vi "HFRR ADV v03 new software.vi"() -> ()   [LabVIEW 2025] (continued)
                frame 126, Default {
                }
              }
            }
          }
          frame #1 {
            w4146 = TRUE ("Visible")
            n3112 = local read "S 91"() -> (w4163:string)
            n3113 = local read "S 90"() -> (w4162:string)
            n3114 = local read "S 88"() -> (w4161:string)
            n3115 = property on="File Path" class="Path"("Caption.Text"=w4162) -> ()  [unwired: 2 in, 2 out]
            n3116 = property on="SrvM CP" class="Bool (strict)"("Boolean Text.Text"=w4161) -> ()  [unwired: 2 in, 2 out]
            n3117 = local read "S 71"() -> (w4156:string)
            n3118 = local read "S 86"() -> (w4158:string)
            n3119 = local read "S 85"() -> (w4159:string)
            n3120 = local read "S 87"() -> (w4157:string)
            n3121 = local read "S 84"() -> (w4160:string)
            n3122 = local read "S 103"() -> (w4145:string)
            n3123 = local read "S 104"() -> (w4144:string)
            n3124 = property on="ENTER THE NEW PASSWORD" class="Str"("Caption.Text"=w4157) -> ()  [unwired: 2 in, 2 out]
            n3125 = property on="Password" class="Str"("Caption.Text"=w4159) -> ()  [unwired: 2 in, 2 out]
            n3126 = property on="ENTER CURRENT PASSWORD" class="Str"("Caption.Text"=w4158) -> ()  [unwired: 2 in, 2 out]
            n3127 = property on="EDIT" class="Bool (strict)"("Boolean Text.Text"=w4156) -> ()  [unwired: 2 in, 2 out]
            n3128 = property on="SAVE" class="Bool (strict)"("Boolean Text.Text"=w4160) -> ()  [unwired: 2 in, 2 out]
            n3129 = Build Array(w4145, w4144) -> (w4143:string[])
            n3130 = property on="Heater Button" class="Bool (strict)"("Strings [4]"=w4143) -> ()  [unwired: 2 in, 2 out]
            n3131 = property on="CH-HUMIDITY WET" class="DigNum (strict)"("Caption.Size to Text?"=w4146) -> ()  [unwired: 2 in, 2 out]
            n3132 = property on="CH-HUMIDITY DRY" class="DigNum (strict)"("Caption.Size to Text?"=w4146) -> ()  [unwired: 2 in, 2 out]
            n3133 = property on="CH-POWER -" class="DigNum (strict)"("Caption.Size to Text?"=w4146) -> ()  [unwired: 2 in, 2 out]
            n3134 = property on="CH-HEATER" class="DigNum (strict)"("Caption.Size to Text?"=w4146) -> ()  [unwired: 2 in, 2 out]
            n3135 = property on="CH-POWER +" class="DigNum (strict)"("Caption.Size to Text?"=w4146) -> ()  [unwired: 2 in, 2 out]
            n3136 = local read "S 92"() -> (w4155:string)
            n3137 = local read "S 93"() -> (w4154:string)
            n3138 = local read "S 105"() -> (w4141:string)
            n3139 = local read "S 106"() -> (w4140:string)
            n3140 = Build Array(w4155, w4154) -> ()  [unwired: 1 out]
            n3141 = Build Array(w4141, w4140) -> (w4142:string[])
            n3142 = local read "S 95"() -> (w4152:string)
            n3143 = local read "S 94"() -> (w4153:string)
            n3144 = local read "bs"() -> (w4168:string)
            n3145 = local read "as"() -> (w4169:string)
            n3146 = property on="Humidity" class="Bool (strict)"("Strings [4]"=w4142) -> ()  [unwired: 2 in, 2 out]
            n3147 = Concatenate Strings(w4168, "\r", w4169) -> ()  [unwired: 1 out]
            n3148 = property on="STROKE GAIN :" class="DigNum (strict)"("Caption.Text"=w4152) -> ()  [unwired: 2 in, 2 out]
            n3149 = property on="DISPLACEMENT :" class="DigNum (strict)"("Caption.Text"=w4153) -> ()  [unwired: 2 in, 2 out]
            n3150 = property on="Rh After" class="DigNum (strict)"("Caption.Size to Text?"=TRUE ("Caption.Size to Text")) -> ()  [unwired: 2 in, 2 out]
            n3151 = local read "S 48"() -> (w4192:string)
            n3152 = local read "S 50"() -> (w4190:string)
            n3153 = local read "S 51"() -> (w4189:string)
            n3154 = local read "S 49"() -> (w4191:string)
            n3155 = local read "S 52"() -> (w4188:string)
            n3156 = local read "as"() -> (w4173:string)
            n3157 = local read "bs"() -> (w4174:string)
            n3158 = local read "S 56"() -> (w4187:string)
            n3159 = local read "S 57"() -> (w4186:string)
            n3160 = local read "S 58"() -> (w4185:string)
            n3161 = local read "S 59"() -> (w4184:string)
            n3162 = property on="OPEN" class="Bool (strict)"("Boolean Text.Text"=w4188) -> ()  [unwired: 2 in, 2 out]
            n3163 = property on="OPEN 1" class="Bool (strict)"("Boolean Text.Text"=w4192) -> ()  [unwired: 2 in, 2 out]
            n3164 = property on="OPEN 2" class="Bool (strict)"("Boolean Text.Text"=w4191) -> ()  [unwired: 2 in, 2 out]
            n3165 = property on="OPEN 3" class="Bool (strict)"("Boolean Text.Text"=w4190) -> ()  [unwired: 2 in, 2 out]
            n3166 = property on="OPEN 4" class="Bool (strict)"("Boolean Text.Text"=w4189) -> ()  [unwired: 2 in, 2 out]
            n3167 = Concatenate Strings(w4174, "\r", w4173) -> ()  [unwired: 1 out]
            n3168 = local read "S 102"() -> (w4147:string)
            n3169 = property on="КОФ1" class="DigNum (strict)"("Caption.Text"=w4187) -> ()  [unwired: 2 in, 2 out]
            n3170 = local read "S 98"() -> (w4151:string)
            n3171 = local read "S 99"() -> (w4150:string)
            n3172 = local read "S 100"() -> (w4149:string)
            n3173 = local read "S 101"() -> (w4148:string)
            n3174 = property on="КОФ2" class="DigNum (strict)"("Caption.Text"=w4186) -> ()  [unwired: 2 in, 2 out]
            n3175 = property on="КОФ3" class="DigNum (strict)"("Caption.Text"=w4185) -> ()  [unwired: 2 in, 2 out]
            n3176 = property on="КОФ4" class="DigNum (strict)"("Caption.Text"=w4184) -> ()  [unwired: 2 in, 2 out]
            n3177 = local read "bs"() -> (w4172:string)
            n3178 = local read "as"() -> (w4171:string)
            n3179 = property on="CH-POWER +" class="DigNum (strict)"("Caption.Text"=w4151) -> ()  [unwired: 2 in, 2 out]
            n3180 = property on="CH-POWER -" class="DigNum (strict)"("Caption.Text"=w4150) -> ()  [unwired: 2 in, 2 out]
            n3181 = property on="CH-HEATER" class="DigNum (strict)"("Caption.Text"=w4149) -> ()  [unwired: 2 in, 2 out]
            n3182 = property on="CH-HUMIDITY DRY" class="DigNum (strict)"("Caption.Text"=w4148) -> ()  [unwired: 2 in, 2 out]
            n3183 = property on="CH-HUMIDITY WET" class="DigNum (strict)"("Caption.Text"=w4147) -> ()  [unwired: 2 in, 2 out]
            n3184 = local read "S 60"() -> (w4183:string)
            n3185 = local read "S 54"() -> (w4193:string)
            n3186 = Concatenate Strings(w4172, "\r", w4171) -> ()  [unwired: 1 out]
            n3187 = Concatenate Strings(w4193, w4183) -> ()  [unwired: 1 out]
            n3188 = local read "S 77"() -> (→"String 43":string)
            n3189 = local read "S 76"() -> (w4166:string)
            n3190 = local read "S 78"() -> (w4165:string)
            n3191 = local read "S 71"() -> (w4177:string)
            n3192 = local read "S 66"() -> (w4182:string)
            n3193 = local read "S 67"() -> (w4181:string)
            n3194 = local read "S 68"() -> (w4180:string)
            n3195 = local read "S 69"() -> (w4179:string)
            n3196 = local read "S 70"() -> (w4178:string)
            n3197 = property on="AIR TEMP" class="DigNum (strict)"("Caption.Text"=w4165) -> ()  [unwired: 2 in, 2 out]
            n3198 = property on="Set Strk" class="DigNum (strict)"("Caption.Text"=w4166) -> ()  [unwired: 2 in, 2 out]
            n3199 = property on="FRIC. FORCE :" class="DigNum (strict)"("Caption.Text"=w4182) -> ()  [unwired: 2 in, 2 out]
            n3200 = property on="TEMPERATURE :" class="DigNum (strict)"("Caption.Text"=w4181) -> ()  [unwired: 2 in, 2 out]
            n3201 = property on="SPEED OUT:" class="DigNum (strict)"("Caption.Text"=w4180) -> ()  [unwired: 2 in, 2 out]
            n3202 = property on="AIR TEMPERATURE :" class="DigNum (strict)"("Caption.Text"=w4179) -> ()  [unwired: 2 in, 2 out]
            n3203 = property on="HUMIDITY:" class="DigNum (strict)"("Caption.Text"=w4178) -> ()  [unwired: 2 in, 2 out]
            n3204 = property on="EDIT" class="Bool (strict)"("Boolean Text.Text"=w4177) -> ()  [unwired: 2 in, 2 out]
            n3205 = local read "S 79"() -> (w4164:string)
          }
          frame #2 {
          }
        }
        n3206 = local write "Lan flag"(10.0 ("Lan flag")) -> ()
      }
      frame Enabled {
      }
    }
    n3207 = Wait (ms)(milliseconds to wait=u32 2000) -> ()  [unwired: 1 out]
    n3208 = local read "Quit"() -> (w3967:bool)
  }
  n3209 = disable-structure shown="Disabled" {
    frame Disabled {
      n3210 = while {
        tunnel: [w4195] -> _
        i -> [w4195]
        stop <- w4194 continue-if-true
        n3211 = Wait (ms)(milliseconds to wait=u32 50) -> ()  [unwired: 1 out]
        n3212 = stacked-sequence {
          frame #0 {
            # "Controls Text color"
            # "Controls BG color"
            n3213 = property on="FILE" class="Str"("Text.Text Colors:Text Color"="SC  Text") -> ()  [unwired: 2 in, 2 out]
            n3214 = property on="Fuel Discription :" class="Str"("Text.Text Colors:Text Color"="SC  Text") -> ()  [unwired: 2 in, 2 out]
            n3215 = property on="tested by" class="Str"("Text.Text Colors:Text Color"="SC  Text") -> ()  [unwired: 2 in, 2 out]
            n3216 = property on="Remarks :" class="Str"("Text.Text Colors:Text Color"="SC  Text") -> ()  [unwired: 2 in, 2 out]
            n3217 = property class="DigNum (strict)"("Numeric Text.Text Colors:BG Color"="NC BG") -> ()  [unwired: 2 in, 2 out]
            n3218 = property class="DigNum (strict)"("Numeric Text.Text Colors:BG Color"="NC BG") -> ()  [unwired: 2 in, 2 out]
            n3219 = property class="DigNum (strict)"("Numeric Text.Text Colors:BG Color"="NC BG") -> ()  [unwired: 2 in, 2 out]
            n3220 = property class="DigNum (strict)"("Numeric Text.Text Colors:BG Color"="NC BG") -> ()  [unwired: 2 in, 2 out]
            n3221 = property class="DigNum (strict)"("Numeric Text.Text Colors:BG Color"="NC BG") -> ()  [unwired: 2 in, 2 out]
            n3222 = property class="DigNum (strict)"("Numeric Text.Text Colors:BG Color"="NC BG") -> ()  [unwired: 2 in, 2 out]
            n3223 = property class="DigNum (strict)"("Numeric Text.Text Colors:BG Color"="NC BG") -> ()  [unwired: 2 in, 2 out]
            n3224 = property class="DigNum (strict)"("Numeric Text.Text Colors:BG Color"="NC BG") -> ()  [unwired: 2 in, 2 out]
            n3225 = property class="DigNum (strict)"("Numeric Text.Text Colors:BG Color"="NC BG") -> ()  [unwired: 2 in, 2 out]
            n3226 = property class="DigNum (strict)"("Numeric Text.Text Colors:BG Color"="NC BG") -> ()  [unwired: 2 in, 2 out]
            n3227 = property class="DigNum (strict)"("Numeric Text.Text Colors:BG Color"="NC BG") -> ()  [unwired: 2 in, 2 out]
            n3228 = property class="DigNum (strict)"("Numeric Text.Text Colors:BG Color"="NC BG") -> ()  [unwired: 2 in, 2 out]
            n3229 = property on="FILE" class="Str"("Text.Text Colors:BG Color"="SC BG 3") -> ()  [unwired: 2 in, 2 out]
            n3230 = property on="Fuel Discription :" class="Str"("Text.Text Colors:BG Color"="SC BG 3") -> ()  [unwired: 2 in, 2 out]
            n3231 = property on="tested by" class="Str"("Text.Text Colors:BG Color"="SC BG 3") -> ()  [unwired: 2 in, 2 out]
            n3232 = property on="Remarks :" class="Str"("Text.Text Colors:BG Color"="SC BG 3") -> ()  [unwired: 2 in, 2 out]
            n3233 = property class="DigNum (strict)"("Numeric Text.Text Colors:Text Color"="NC Text") -> ()  [unwired: 2 in, 2 out]
            n3234 = property class="DigNum (strict)"("Numeric Text.Text Colors:Text Color"="NC Text") -> ()  [unwired: 2 in, 2 out]
            n3235 = property class="DigNum (strict)"("Numeric Text.Text Colors:Text Color"="NC Text") -> ()  [unwired: 2 in, 2 out]
            n3236 = property class="DigNum (strict)"("Numeric Text.Text Colors:Text Color"="NC Text") -> ()  [unwired: 2 in, 2 out]
            n3237 = property class="DigNum (strict)"("Numeric Text.Text Colors:Text Color"="NC Text") -> ()  [unwired: 2 in, 2 out]
            n3238 = property class="DigNum (strict)"("Numeric Text.Text Colors:Text Color"="NC Text") -> ()  [unwired: 2 in, 2 out]
            n3239 = property class="DigNum (strict)"("Numeric Text.Text Colors:Text Color"="NC Text") -> ()  [unwired: 2 in, 2 out]
            n3240 = property class="DigNum (strict)"("Numeric Text.Text Colors:Text Color"="NC Text") -> ()  [unwired: 2 in, 2 out]
            n3241 = property class="DigNum (strict)"("Numeric Text.Text Colors:Text Color"="NC Text") -> ()  [unwired: 2 in, 2 out]
            n3242 = property class="DigNum (strict)"("Numeric Text.Text Colors:Text Color"="NC Text") -> ()  [unwired: 2 in, 2 out]
            n3243 = property class="DigNum (strict)"("Numeric Text.Text Colors:Text Color"="NC Text") -> ()  [unwired: 2 in, 2 out]
            n3244 = property class="DigNum (strict)"("Numeric Text.Text Colors:Text Color"="NC Text") -> ()  [unwired: 2 in, 2 out]
            n3245 = property class="DigNum (strict)"("Numeric Text.Text Colors:Text Color"="NI Text  2") -> ()  [unwired: 2 in, 2 out]
            n3246 = property class="DigNum (strict)"("Numeric Text.Text Colors:Text Color"="NI Text  2") -> ()  [unwired: 2 in, 2 out]
            n3247 = property class="DigNum (strict)"("Numeric Text.Text Colors:Text Color"="NI Text  2") -> ()  [unwired: 2 in, 2 out]
            n3248 = property class="DigNum (strict)"("Numeric Text.Text Colors:Text Color"="NI Text  2") -> ()  [unwired: 2 in, 2 out]
            n3249 = property class="DigNum (strict)"("Numeric Text.Text Colors:Text Color"="NI Text  2") -> ()  [unwired: 2 in, 2 out]
            n3250 = property class="DigNum (strict)"("Numeric Text.Text Colors:Text Color"="NI Text  2") -> ()  [unwired: 2 in, 2 out]
            n3251 = property class="DigNum (strict)"("Numeric Text.Text Colors:Text Color"="NI Text  2") -> ()  [unwired: 2 in, 2 out]
            n3252 = property class="DigNum (strict)"("Numeric Text.Text Colors:Text Color"="NI Text  2") -> ()  [unwired: 2 in, 2 out]
            n3253 = property class="DigNum (strict)"("Numeric Text.Text Colors:Text Color"="NI Text  2") -> ()  [unwired: 2 in, 2 out]
            n3254 = property class="DigNum (strict)"("Numeric Text.Text Colors:Text Color"="NI Text  2") -> ()  [unwired: 2 in, 2 out]
            n3255 = property class="DigNum (strict)"("Numeric Text.Text Colors:Text Color"="NI Text  2") -> ()  [unwired: 2 in, 2 out]
            n3256 = property class="DigNum (strict)"("Numeric Text.Text Colors:Text Color"="NI Text  2") -> ()  [unwired: 2 in, 2 out]
            n3257 = property class="DigNum (strict)"("Numeric Text.Text Colors:Text Color"="NI Text  2") -> ()  [unwired: 2 in, 2 out]
            n3258 = property class="DigNum (strict)"("Numeric Text.Text Colors:Text Color"="NI Text  2") -> ()  [unwired: 2 in, 2 out]
            n3259 = property class="DigNum (strict)"("Numeric Text.Text Colors:Text Color"="NI Text  2") -> ()  [unwired: 2 in, 2 out]
            n3260 = property on="Coefficient Of Friction" class="XYGraph (strict)"("Plot Area:Colors:FG Color"="GFG  2", "Plot Area:Colors:BG Color"="GBG   2") -> ()  [unwired: 2 in, 2 out]
            n3261 = property on="Humidity ( %RH )" class="XYGraph (strict)"("Plot Area:Colors:FG Color"="GFG  2", "Plot Area:Colors:BG Color"="GBG   2") -> ()  [unwired: 2 in, 2 out]
            n3262 = property on="Air Temperature  ( °C )" class="XYGraph (strict)"("Plot Area:Colors:FG Color"="GFG  2", "Plot Area:Colors:BG Color"="GBG   2") -> ()  [unwired: 2 in, 2 out]
            n3263 = property on="Sample Temperature ( °C )" class="XYGraph (strict)"("Plot Area:Colors:FG Color"="GFG  2", "Plot Area:Colors:BG Color"="GBG   2") -> ()  [unwired: 2 in, 2 out]
            n3264 = property class="DigNum (strict)"("Numeric Text.Text Colors:BG Color"="NI BG 2") -> ()  [unwired: 2 in, 2 out]
            n3265 = property class="DigNum (strict)"("Numeric Text.Text Colors:BG Color"="NI BG 2") -> ()  [unwired: 2 in, 2 out]
            n3266 = property class="DigNum (strict)"("Numeric Text.Text Colors:BG Color"="NI BG 2") -> ()  [unwired: 2 in, 2 out]
            n3267 = property class="DigNum (strict)"("Numeric Text.Text Colors:BG Color"="NI BG 2") -> ()  [unwired: 2 in, 2 out]
            n3268 = property class="DigNum (strict)"("Numeric Text.Text Colors:BG Color"="NI BG 2") -> ()  [unwired: 2 in, 2 out]
            n3269 = property class="DigNum (strict)"("Numeric Text.Text Colors:BG Color"="NI BG 2") -> ()  [unwired: 2 in, 2 out]
            n3270 = property class="DigNum (strict)"("Numeric Text.Text Colors:BG Color"="NI BG 2") -> ()  [unwired: 2 in, 2 out]
            n3271 = property class="DigNum (strict)"("Numeric Text.Text Colors:BG Color"="NI BG 2") -> ()  [unwired: 2 in, 2 out]
            n3272 = property class="DigNum (strict)"("Numeric Text.Text Colors:BG Color"="NI BG 2") -> ()  [unwired: 2 in, 2 out]
            n3273 = property class="DigNum (strict)"("Numeric Text.Text Colors:BG Color"="NI BG 2") -> ()  [unwired: 2 in, 2 out]
            n3274 = property class="DigNum (strict)"("Numeric Text.Text Colors:BG Color"="NI BG 2") -> ()  [unwired: 2 in, 2 out]
            n3275 = property class="DigNum (strict)"("Numeric Text.Text Colors:BG Color"="NI BG 2") -> ()  [unwired: 2 in, 2 out]
            n3276 = property class="DigNum (strict)"("Numeric Text.Text Colors:BG Color"="NI BG 2") -> ()  [unwired: 2 in, 2 out]
            n3277 = property class="DigNum (strict)"("Numeric Text.Text Colors:BG Color"="NI BG 2") -> ()  [unwired: 2 in, 2 out]
            n3278 = property class="DigNum (strict)"("Numeric Text.Text Colors:BG Color"="NI BG 2") -> ()  [unwired: 2 in, 2 out]
            n3279 = property class="Bool"("Colors [4]"="Boolean BC T & BG") -> ()  [unwired: 2 in, 2 out]
            n3280 = property on="Save & Continue" class="Bool (strict)"("Colors [4]"="Boolean BC T & BG") -> ()  [unwired: 2 in, 2 out]
            n3281 = property on="Heater Button" class="Bool (strict)"("Colors [4]"="Boolean BC T & BG") -> ()  [unwired: 2 in, 2 out]
            n3282 = property class="Bool"("Colors [4]"="Boolean BC T & BG") -> ()  [unwired: 2 in, 2 out]
            n3283 = property on="Humidity" class="Bool (strict)"("Colors [4]"="Boolean BC T & BG") -> ()  [unwired: 2 in, 2 out]
            n3284 = property class="Bool (strict)"("Colors [4]"="Boolean BC T & BG") -> ()  [unwired: 2 in, 2 out]
            n3285 = property on="RUN" class="Bool (strict)"("Colors [4]"="Boolean BC T & BG") -> ()  [unwired: 2 in, 2 out]
            n3286 = property on="trip1 8" class="Bool (strict)"("Colors [4]"="Boolean BC T & BG") -> ()  [unwired: 2 in, 2 out]
            n3287 = property class="Bool"("Colors [4]"="Boolean BC T & BG") -> ()  [unwired: 2 in, 2 out]
            n3288 = property class="Bool (strict)"("Colors [4]"="Boolean BC T & BG") -> ()  [unwired: 2 in, 2 out]
            n3289 = property on="OPEN 1" class="Bool (strict)"("Colors [4]"="Boolean BC T & BG 2") -> ()  [unwired: 2 in, 2 out]
            n3290 = property on="OPEN 2" class="Bool (strict)"("Colors [4]"="Boolean BC T & BG 2") -> ()  [unwired: 2 in, 2 out]
            n3291 = property on="OPEN 3" class="Bool (strict)"("Colors [4]"="Boolean BC T & BG 2") -> ()  [unwired: 2 in, 2 out]
            n3292 = property on="OPEN 4" class="Bool (strict)"("Colors [4]"="Boolean BC T & BG 2") -> ()  [unwired: 2 in, 2 out]
            n3293 = property on="OPEN" class="Bool (strict)"("Colors [4]"="Boolean BC T & BG 2") -> ()  [unwired: 2 in, 2 out]
            n3294 = property on="rstv2" class="Bool"("Colors [4]"="Boolean BC T & BG 2") -> ()  [unwired: 2 in, 2 out]
            n3295 = property on="RST CP" class="Bool"("Colors [4]"="Boolean BC T & BG 2") -> ()  [unwired: 2 in, 2 out]
            n3296 = property on="RSTV1 3" class="Bool"("Colors [4]"="Boolean BC T & BG 2") -> ()  [unwired: 2 in, 2 out]
            n3297 = property on="RSTV1 2" class="Bool"("Colors [4]"="Boolean BC T & BG 2") -> ()  [unwired: 2 in, 2 out]
          }
          frame #1 {
          }
        }
        n3298 = local read "Quit"() -> (w4194:bool)
      }
    }
    frame Enabled {
    }
  }
  n3299 = while {
    shift-right: [w4212] -> _
    shift-left: _ -> [w4213]
    shift-right: [w4210] -> _
    shift-left: T14 {"Read Heave and Surge"="", "Bytes at Heave Port"=0.0, "Heave and Surge COM Port:"="COM9", "Com Port 2"="COM7", "Residual Due"="", "Heave COM Status 2"=TRUE, "Heave COM Status"=TRUE, "Port 2"=TRUE, "Sway PPR"=6400.0, "Surge PPR"=6400.0, "Heave PPR"=6400.0, "Sway Pitch"=2.0, "Surge Pitch"=3.0, "Heave Pitch"=4.0, "Sway Pulses/mm"=320.0, "Surge Pulses/mm"=1600.0, "Heave Pulses/mm"=1600.0, "inner loop"=0.0, "Read Heave and Surge 2"="", "String 36"="", "Write S"=FALSE, "WriteCC1"=[""], "Heave COM Loop"=0, "LastCom"="", "EXIT"=FALSE, "Error Heave"={"status"=TRUE, "code"=-1073807343, "source"=""}} -> [w4209]
    shift-right: [w4207] -> _
    shift-left: enum16{"init", "MAIN", "Panel Close"}."init" -> [w4208]
    stop <- w4211 stop-if-true
    n3300 = case shown="\"init\"" w4208 {
      tunnel: w4213 -> [w4227 w4242 w4312 w4314]
      tunnel: [w4221 w4260 w4312 w4314] -> w4212
      tunnel: [_ _ TRUE _] -> w4211
      tunnel: [w4217 w4257 w4310 w4313] -> w4210
      tunnel: w4209 -> [w4224 w4241 w4310 w4313]
      tunnel: [enum16{"init", "MAIN", "Panel Close"}."MAIN" w4235 _ _] -> w4207
      frame "init" {
        n3301 = Bundle By Name(cluster=w4224, "Heave and Surge COM Port:"="C3 :") -> (w4223:T14)
        n3302 = call "Instrument fgv.vi"("Enum"=T24."INIT", "error in (no error) 2"=w4227, "INPUT"=w4223) -> ("error"=w4225:errorcluster, "output"=w4220:T14)  [unwired: 6 in, 1 out]
        n3303 = case shown="No Error" w4225 {
          selector: w4225 -> [w4229 _]
          tunnel: [w4229 w4233] -> w4221
          tunnel: w4220 -> [w4228 w4231]
          tunnel: [w4228 w4230] -> w4218
          frame No Error {
          }
          frame Error {
            n3304 = call "Instrument fgv.vi"("Enum"=T24."ERROR INIT", "INPUT"=w4231) -> ("error"=w4234:errorcluster, "output"=w4230:T14)  [unwired: 7 in, 1 out]
            n3305 = call <vilib>:"Clear Errors.vi"("error in (no error)"=w4234) -> ("error out"=w4233:errorcluster)  [unwired: 5 in, 1 out]
          }
        }
        n3306 = local read "LastCom"() -> (w4216:string)
        n3307 = Unbundle By Name(w4218) -> ("Heave COM Status 2"=→"COM Status" →"Instrument Status":bool, "Error Heave"=→"Error":errorcluster)  [unwired: 1 out]
        n3308 = Bundle By Name(cluster=w4218, "LastCom"=w4216) -> (w4217:T14)
      }
      frame "MAIN" {
        n3309 = Unbundle By Name(w4241) -> ("Com Port 2"=w4262:refnum<visa-resource-name>)
        n3310 = local write "Com Port 4"(w4262) -> ()
        n3311 = local read "C3 :"() -> (w4239:refnum<visa-resource-name>)
        n3312 = Divide(x="Heave PPR", y="Heave Pitch") -> (x/y=→"Heave Pulses/mm":dbl)
        n3313 = Bundle By Name(cluster=w4241, "Heave and Surge COM Port:"=w4239) -> (w4240:T14)
        n3314 = Equal?(x=w4262, y=w4239) -> (x = y?=w4261:bool)
        n3315 = Divide(x="Sway PPR", y="Sway Pitch") -> (x/y=→"Sway Pulses/mm":dbl)
        n3316 = case shown="False" w4261 {
          tunnel: [w4266 w4283] -> w4260
          tunnel: w4242 -> [w4267 w4289]
          tunnel: w4240 -> [w4265 w4287]
          tunnel: [w4264 w4282] -> w4257
          frame False {
            n3317 = call <vilib>:"Clear Errors.vi"("error in (no error)"=w4267) -> ("error out"=w4263:errorcluster)  [unwired: 5 in, 1 out]
            n3318 = call "Instrument fgv.vi"("Enum"=T24."ERROR INIT", "error in (no error) 2"=w4263, "INPUT"=w4265) -> ("error"=w4269:errorcluster, "output"=w4264:T14)  [unwired: 6 in, 1 out]
            n3319 = call <vilib>:"Clear Errors.vi"("error in (no error)"=w4269) -> ("error out"=w4266:errorcluster)  [unwired: 5 in, 1 out]
          }
          frame True {
            n3320 = call "Instrument fgv.vi"("Enum"=T24."READ", "error in (no error) 2"=w4289, "INPUT"=w4287) -> ("error"=w4288:errorcluster, "output"=w4279:T14)  [unwired: 6 in, 1 out]
            n3321 = Bundle By Name(cluster=w4279, "String 36"="String 11") -> (w4278:T14)
            n3322 = case shown="True" "Write S" {
              selector: "Write S" -> [_ w4309]
              tunnel: w4288 -> [w4302 w4308]
              tunnel: [w4302 w4307] -> w4275
              tunnel: w4278 -> [w4301 w4304]
              tunnel: [w4301 w4303] -> w4274
              frame False {
              }
              frame True {
                n3323 = Not(x=w4309) -> (.not. x?=w4305:bool)
                n3324 = local write "Write S"(w4305) -> ()
                n3325 = call "Instrument fgv.vi"("Enum"=T24."MANUAL WRITE", "error in (no error) 2"=w4308, "INPUT"=w4304) -> ("error"=w4307:errorcluster, "output"=w4303:T14)  [unwired: 6 in, 1 out]
              }
            }
            n3326 = Array Size(array="WriteHumidity") -> (size(s)=w4272:i32)
            n3327 = Greater Than 0?(x=w4272) -> (x > 0?=w4270:bool)
            n3328 = call "Instrument fgv.vi"("Enum"=T24."WRITE", "error in (no error) 2"=w4275, "WriteCC1"="WriteHumidity", "INPUT"=w4274) -> ("error"=w4285:errorcluster, "WriteCC1 2"=w4273:string[], "output"=w4284:T14)  [unwired: 5 in]
            n3329 = case shown="True" w4270 {
              tunnel: w4273 -> [_ w4291]
              frame False {
              }
              frame True {
                n3330 = local write "WriteHumidity"(w4291) -> ()
              }
            }
            n3331 = case shown="Error" w4285 {
              selector: w4285 -> [w4292 w4295]
              tunnel: w4284 -> [w4293 w4300]
              tunnel: [w4293 w4299] -> w4282
              tunnel: [w4292 w4297] -> w4283
              frame No Error {
              }
              frame Error {
                n3332 = call <vilib>:"Clear Errors.vi"("error in (no error)"=w4295) -> ("error out"=w4294:errorcluster)  [unwired: 5 in, 1 out]
                n3333 = call "Instrument fgv.vi"("Enum"=T24."ERROR INIT", "error in (no error) 2"=w4294, "INPUT"=w4300) -> ("error"=w4298:errorcluster, "output"=w4299:T14)  [unwired: 6 in, 1 out]
                n3334 = call <vilib>:"Clear Errors.vi"("error in (no error)"=w4298) -> ("error out"=w4297:errorcluster)  [unwired: 5 in, 1 out]
              }
            }
            n3335 = Unbundle By Name(w4282) -> ("LastCom"=→"LastCom":string, "Read Heave and Surge"=→"Read Humidity":string)
          }
        }
        n3336 = Divide(x="Surge PPR", y="Surge Pitch") -> (x/y=→"Surge Pulses/mm":dbl)
        n3337 = Unbundle By Name(w4257) -> ("Heave COM Status 2"=w4259:bool, "Heave COM Status"=w4258:bool, "Error Heave"=w4255:errorcluster, "Bytes at Heave Port"=→"Bytes at Humidity Port":dbl)
        n3338 = Unbundle By Name(w4255) -> ("status"=→"Humidity Port":bool)
        n3339 = Not(x=w4258) -> (.not. x?=w4243:bool)
        n3340 = local write "Error"(w4255) -> ()
        n3341 = Not(x=w4259) -> (.not. x?=w4244:bool)
        n3342 = local write "Instrument Status"(w4243) -> ()
        n3343 = local write "COM Status"(w4244) -> ()
        n3344 = local read "Quit"() -> (w4236:bool)
        n3345 = Select(t=enum16{"init", "MAIN", "Panel Close"}."Panel Close", s=w4236, f=enum16{"init", "MAIN", "Panel Close"}."MAIN") -> (s? t:f=w4235:enum16{"init", "MAIN", "Panel Close"})
      }
      frame "Panel Close" {
      }
      frame Default {
      }
    }
  }
  n3346 = while {
    stop <- w4340 stop-if-true
    n3347 = local read "Read Humidity"() -> (w4321:string)
    n3348 = call <vilib>:"High Resolution Polling Wait.vi"("seconds to wait"=0.1) -> ()  [unwired: 10 in, 1 out]
    n3349 = Spreadsheet String To Array(delimiter (Tab)=",", format string="", spreadsheet string=w4321, array type (2D Dbl)=string[] []) -> (array=w4335:string[])
    n3350 = for {
      tunnel: w4335 -> [w4345] mode=indexing
      tunnel: string[] ["STATE;", "SET;", "RH;", "T;", "AMB_RH;", "AMB_T;", "PUMP;", "FAN_IN;", "FAN_OUT;", "DEHUM;", "CURRENT;", "STALL;"] -> [w4344] mode=indexing
      tunnel: [w4343] -> w4334 mode=indexing
      n3351 = Match Pattern(string=w4345, regular expression=w4344) -> (after substring=w4343:string)  [unwired: 1 in, 3 out]
    }
    n3352 = Index Array(array=w4334) -> (element #1=→"STATE :":string, element #2=→"SET :":string, element #3=w4323:string, element #4=→"T :":string, element #5=w4320:string, element #6=→"AMB_T :":string, element #7=→"PUMP :":string, element #8=→"FAN_IN :":string, element #9=→"FAN_OUT :":string, element #10=→"DEHUM :":string, element #11=→"CURRENT :":string, element #12=→"STALL :":string)  [unwired: 12 in]
    "RH :" <- w4323
    "AMB_RH :" <- w4320
    n3353 = Fract/Exp String To Number(string=w4323) -> (number=w4315:dbl)  [unwired: 3 in, 1 out]
    n3354 = Fract/Exp String To Number(string=w4320) -> (number=w4319:dbl)  [unwired: 3 in, 1 out]
    n3355 = local write "Ambient Humidity :"(w4319) -> ()
    n3356 = Equal?(x=w4315, y=0.0) -> (x = y?=w4317:bool)
    n3357 = case shown="True" w4317 {
      tunnel: [w4341 w4342] -> w4316
      tunnel: w4315 -> [w4341 _]
      frame False {
        (unwired) 0.0
        "Humidity temp" <- w4341
      }
      frame True {
        n3358 = local read "Humidity temp"() -> (w4342:dbl)
      }
    }
    "RH Numeric:" <- w4316
    n3359 = local read "Quit"() -> (w4340:bool)
  }
  n3360 = disable-structure shown="Disabled" {
    frame Disabled {
      n3361 = while {
        tunnel: [w4579] -> _
        i -> [w4579]
        stop <- w4576 stop-if-true
        n3362 = local read "powstat"() -> (w4577:bool)
        n3363 = case shown="True" w4577 {
          frame False {
          }
          frame True {
            n3364 = local read "RUN"() -> (w4580:bool)
            n3365 = case shown="True" w4580 {
              frame False {
                w4610 = 65.0 ("y")
                n3366 = local read "Set Hz"() -> (w4638:dbl)
                n3367 = local read "NORMAL LOAD"() -> (w4639:dbl)
                n3368 = Multiply(x=w4638, y=60.0) -> (x*y=w4645:dbl)
                n3369 = Multiply(x=1.2 ("y"), y=0.949) -> (x*y=w4614:dbl)
                n3370 = Multiply(x=1.2 ("y"), y=0.8166) -> (x*y=w4618:dbl)
                n3371 = Multiply(x=1.2 ("y"), y=0.851) -> (x*y=w4613:dbl)
                n3372 = local read "FF 2"() -> (w4637:dbl)
                n3373 = Absolute Value(x=w4645) -> (abs(x)=w4643:dbl)
                n3374 = case shown="13.." w4637 {
                  tunnel: [1 2 3] -> w4635
                  frame 0..10, Default {
                    # "Normal"
                  }
                  frame 11, 12 {
                  }
                  frame 13.. {
                  }
                }
                "FF STATE" <- w4635
                n3375 = local read "TEMP"() -> (w4598:dbl)
                n3376 = local read item#-1() -> (w4612)
                n3377 = Less?(x=w4612, y=w4618) -> (x < y?=w4615:bool)
                n3378 = In Range and Coerce(upper limit=w4614, x=w4612, lower limit=w4613) -> (In Range?=w4616:bool)  [unwired: 1 out]
                n3379 = case shown="3601.." w4643 {
                  tunnel: [1 2 3] -> w4641
                  frame 0..3000, Default {
                    # "Normal"
                  }
                  frame 3001..3600 {
                  }
                  frame 3601.. {
                  }
                }
                n3380 = case shown="11.." w4639 {
                  tunnel: [1 3] -> w4640
                  frame 1..10, Default {
                  }
                  frame 11.. {
                  }
                }
                "NL STATE" <- w4640
                n3381 = Multiply(x=1.2 ("y"), y=0.95) -> (x*y=w4628:dbl)
                n3382 = Multiply(x=w4610, y=0.954) -> (x*y=w4602:dbl)
                n3383 = Or(x=w4615, y=w4616) -> (x .or. y?=w4617:bool)
                n3384 = Greater Or Equal?(x=w4612, y=w4628) -> (x >= y?=w4625:bool)
                n3385 = Multiply(x=w4610, y=0.99) -> (x*y=w4599:dbl)
                n3386 = Greater Or Equal?(x=w4598, y=w4599) -> (x >= y?=w4604:bool)
                n3387 = Greater Or Equal?(x=w4598, y=w4602) -> (x >= y?=w4601:bool)
                n3388 = case shown="0, 1, Default" w4612 {
                  tunnel: [1 3] -> w4629
                  frame 0, 1, Default {
                  }
                  frame 2.. {
                  }
                }
                n3389 = case shown="True" w4625 {
                  tunnel: [1 3] -> w4630
                  frame False {
                  }
                  frame True {
                  }
                }
                n3390 = case shown="True" w4617 {
                  tunnel: [1 2] -> w4631
                  frame False {
                  }
                  frame True {
                  }
                }
                n3391 = case shown="..0" w4598 {
                  tunnel: [2 3 3 1] -> w4605
                  frame 61, 62 {
                  }
                  frame 63.. {
                  }
                  frame ..0 {
                  }
                  frame 10..60, Default {
                  }
                }
                n3392 = case shown="True" w4604 {
                  tunnel: [1 3] -> w4606
                  frame False {
                  }
                  frame True {
                  }
                }
                n3393 = Number To Decimal String(number=w4641) -> (decimal integer string=w4642:string)  [unwired: 1 in]
                n3394 = case shown="True" w4601 {
                  tunnel: [1 2] -> w4607
                  frame False {
                  }
                  frame True {
                  }
                }
                n3395 = Number To Decimal String(number=1) -> (decimal integer string=→"Air temp":string)  [unwired: 1 in]
                n3396 = Number To Decimal String(number=w4635) -> (decimal integer string=→"ff_st":string)  [unwired: 1 in]
                n3397 = local write "sp_st"(w4642) -> ()
                n3398 = Number To Decimal String(number=w4640) -> (decimal integer string=→"nl_st":string)  [unwired: 1 in]
                n3399 = Build Array(w4605, w4606, w4607) -> (w4608:i32[])
                n3400 = Build Array(w4629, w4630, w4631) -> (w4632:i32[])
                n3401 = Array Max & Min(array=w4608) -> (max value=w4609:i32)  [unwired: 3 out]
                n3402 = Array Max & Min(array=w4632) -> (max value=w4633:i32)  [unwired: 3 out]
                n3403 = Number To Decimal String(number=w4609) -> (decimal integer string=w4597:string)  [unwired: 1 in]
                n3404 = Number To Decimal String(number=w4633) -> (decimal integer string=→"Stroke Ln 2":string)  [unwired: 1 in]
                n3405 = local write "temp_st"(w4597) -> ()
              }
              frame True {
                w4695 = 65.0 ("y")
                # "Healthy -1\nWarning -2\nError -3"
                n3406 = local read "TEMP"() -> (w4706:dbl)
                n3407 = local read "NORMAL LOAD"() -> (w4710:dbl)
                n3408 = local read "Set Hz"() -> (w4708:dbl)
                n3409 = Multiply(x=1.2 ("y"), y=0.949) -> (x*y=w4690:dbl)
                n3410 = Multiply(x=1.2 ("y"), y=0.8166) -> (x*y=w4686:dbl)
                n3411 = Multiply(x=1.2 ("y"), y=0.851) -> (x*y=w4691:dbl)
                n3412 = Multiply(x=w4695, y=0.954) -> (x*y=w4702:dbl)
                n3413 = Multiply(x=w4695, y=0.99) -> (x*y=w4705:dbl)
                n3414 = Greater Or Equal?(x=w4706, y=w4705) -> (x >= y?=w4700:bool)
                n3415 = Multiply(x=w4708, y=60.0) -> (x*y=w4714:dbl)
                n3416 = Greater Or Equal?(x=w4706, y=w4702) -> (x >= y?=w4703:bool)
                n3417 = local read "FF 2"() -> (w4709:dbl)
                n3418 = local read item#-1() -> (w4692)
                n3419 = Less?(x=w4692, y=w4686) -> (x < y?=w4689:bool)
                n3420 = In Range and Coerce(upper limit=w4690, x=w4692, lower limit=w4691) -> (In Range?=w4688:bool)  [unwired: 1 out]
                n3421 = Absolute Value(x=w4714) -> (abs(x)=w4712:dbl)
                n3422 = case shown="63.." w4706 {
                  tunnel: [2 3 3 1] -> w4699
                  frame 61, 62 {
                  }
                  frame 63.. {
                  }
                  frame ..0 {
                  }
                  frame 10..60, Default {
                  }
                }
                n3423 = case shown="True" w4700 {
                  tunnel: [1 3] -> w4698
                  frame False {
                  }
                  frame True {
                  }
                }
                n3424 = case shown="True" w4703 {
                  tunnel: [1 2] -> w4697
                  frame False {
                  }
                  frame True {
                  }
                }
                n3425 = Multiply(x=1.2 ("y"), y=0.95) -> (x*y=w4676:dbl)
                n3426 = case shown="1..10, Default" w4710 {
                  tunnel: [1 3] -> w4717
                  frame 1..10, Default {
                  }
                  frame 11.. {
                  }
                }
                n3427 = case shown="0..10, Default" w4709 {
                  tunnel: [1 2 3] -> w4716
                  frame 0..10, Default {
                  }
                  frame 11, 12 {
                  }
                  frame 13.. {
                  }
                }
                n3428 = case shown="3601.." w4712 {
                  tunnel: [1 2 3] -> w4711
                  frame 0..3000, Default {
                    # "Normal"
                  }
                  frame 3001..3600 {
                  }
                  frame 3601.. {
                  }
                }
                n3429 = Or(x=w4689, y=w4688) -> (x .or. y?=w4687:bool)
                n3430 = Greater Or Equal?(x=w4692, y=w4676) -> (x >= y?=w4679:bool)
                n3431 = case shown="0, 1, Default" w4692 {
                  tunnel: [1 3] -> w4675
                  frame 0, 1, Default {
                  }
                  frame 2.. {
                  }
                }
                n3432 = case shown="True" w4679 {
                  tunnel: [1 3] -> w4674
                  frame False {
                  }
                  frame True {
                  }
                }
                n3433 = case shown="True" w4687 {
                  tunnel: [1 2] -> w4673
                  frame False {
                  }
                  frame True {
                  }
                }
                n3434 = Build Array(w4699, w4698, w4697) -> (w4696:i32[])
                n3435 = Number To Decimal String(number=w4711) -> (decimal integer string=→"sp_st":string)  [unwired: 1 in]
                n3436 = Array Max & Min(array=w4696) -> (max value=w4693:i32)  [unwired: 3 out]
                "TEMP STATE" <- w4693
                n3437 = Number To Decimal String(number=w4717) -> (decimal integer string=w4720:string)  [unwired: 1 in]
                n3438 = Number To Decimal String(number=w4716) -> (decimal integer string=w4718:string)  [unwired: 1 in]
                n3439 = Number To Decimal String(number=w4693) -> (decimal integer string=→"temp_st":string)  [unwired: 1 in]
                n3440 = Build Array(w4675, w4674, w4673) -> (w4672:i32[])
                n3441 = local write "nl_st"(w4720) -> ()
                n3442 = local write "ff_st"(w4718) -> ()
                n3443 = Number To Decimal String(number=1) -> (decimal integer string=w4715:string)  [unwired: 1 in]
                n3444 = Array Max & Min(array=w4672) -> (max value=w4671:i32)  [unwired: 3 out]
                n3445 = local write "Air temp"(w4715) -> ()
                n3446 = Number To Decimal String(number=w4671) -> (decimal integer string=w4670:string)  [unwired: 1 in]
                n3447 = local write "Stroke Ln 2"(w4670) -> ()
              }
            }
            n3448 = local read "Stroke Ln 2"() -> (w4582:string)
            n3449 = local read "nl_st"() -> (w4588:string)
            n3450 = local read "ff_st"() -> (w4585:string)
            n3451 = local read "sp_st"() -> (w4586:string)
            n3452 = local read "temp_st"() -> (w4587:string)
            n3453 = local read "Air temp"() -> (w4581:string)
            n3454 = Replace Array Subset(array="in", new element #1=w4588, index #1=1 ("index"), new element #2=w4585, index #2=2 ("index"), new element #3=w4587, index #3=3 ("index"), new element #4=w4586, index #4=4 ("index"), new element #5=w4582, index #5=5 ("index"), new element #6=w4581, index #6=6 ("index"), new element #7="Sensor State" ("new element/subarray"), index #7=0 ("index")) -> (→"out":string[])
          }
        }
        n3455 = Wait (ms)(milliseconds to wait=u32 10) -> ()  [unwired: 1 out]
        n3456 = local read "Quit"() -> (w4576:bool)
      }
      n3457 = while {
        stop <- w4551 stop-if-true
        n3458 = local read "run replace"() -> (w4553:bool)
        n3459 = Wait (ms)(milliseconds to wait=u32 100) -> ()  [unwired: 1 out]
        n3460 = Equal?(x="FLAG 2", y=0.0) -> (x = y?=w4554:bool)
        n3461 = case shown="True" w4554 {
          frame False {
          }
          frame True {
            n3462 = local write "FLAG 2"(100.0 ("FLAG 2")) -> ()
            n3463 = call <vilib>:"Read Characters From File.vi"("file path (dialog if empty)"=path "C:/LAB-IQ-NXT/WO 2449 TT.sig", "convert eol? (no:F)"=FALSE ("append to file? (new file:F)")) -> ("character string"=w4557:string)  [unwired: 4 in, 3 out]
            n3464 = call <vilib>:"Read Characters From File.vi"("file path (dialog if empty)"=path "C:/LAB-IQ-NXT/WO 2449 TRH.sig", "convert eol? (no:F)"=FALSE ("append to file? (new file:F)")) -> ("character string"=w4558:string)  [unwired: 4 in, 3 out]
            n3465 = Decimal String To Number(string=w4557) -> (number=w4559:i32)  [unwired: 2 in, 1 out]
            n3466 = local write "Total No. of Tests"(w4559) -> ()
            n3467 = Decimal String To Number(string=w4558) -> (number=w4562:i32)  [unwired: 2 in, 1 out]
            n3468 = local write "SEN.RUN HRS"(w4562) -> ()
          }
        }
        n3469 = case shown="True" w4553 {
          frame False {
          }
          frame True {
            n3470 = Equal?(x="FLAG 4", y=0.0) -> (x = y?=w4566:bool)
            n3471 = case shown="False" w4566 {
              frame False {
                n3472 = Get Date/Time In Seconds() -> (seconds since 1Jan1904=w4572:timestamp)
                n3473 = local read "START 3"() -> (w4570:dbl)
                n3474 = To Double Precision Float(number=w4572) -> (double precision float=w4571:dbl)
                n3475 = Subtract(x=w4571, y=w4570) -> (x-y=→"SENSOR TIME":dbl)
              }
              frame True {
                n3476 = Get Date/Time In Seconds() -> (seconds since 1Jan1904=w4574:timestamp)
                n3477 = local write "FLAG 4"(100.0 ("FLAG")) -> ()
                n3478 = To Double Precision Float(number=w4574) -> (double precision float=→"START 3":dbl)
              }
            }
          }
        }
        n3479 = local read "Quit"() -> (w4551:bool)
      }
      n3480 = while {
        shift-right: [w4351] -> _
        shift-left: _ -> [w4352]
        tunnel: [w4347] -> _
        i -> [w4347]
        stop <- w4346 stop-if-true
        n3481 = Wait (ms)(milliseconds to wait=u32 50 ("Refresh Rate (ms)")) -> ()  [unwired: 1 out]
        n3482 = local read "Json End Flg"() -> (w4348:bool)
        n3483 = Not(x="Upld AR 2") -> ()  [unwired: 1 out]
        n3484 = local read "Upld AR 2"() -> (w4349:bool)
        n3485 = call "Elapsed Time9"("Time Target (s)"="Sen.Upload Rate (s)", "Reset"=FALSE, "Auto Reset"=TRUE) -> ("Time has Elapsed"=w4358:bool)  [unwired: 9 in, 7 out]
        n3486 = Or(x=w4358, y=w4348) -> (x .or. y?=w4354:bool)
        n3487 = case shown="True" w4354 {
          frame False {
          }
          frame True {
            w4450 = "\"SensorName\":\"" ("string")
            w4420 = " \"},{"
            w4445 = "\",\"SensorState\":\""
            w4447 = "\",\"SensorModelNumber\":\"" ("string")
            w4446 = "\",\"SensorRuntimeHours\":\"" ("string")
            n3488 = local read "model num"() -> (w4444:string[])
            n3489 = local read "Sensor name"() -> (w4463:string[])
            n3490 = local read "run"() -> (w4434:string[])
            n3491 = local read "SENSOR TIME"() -> (w4390:dbl)
            n3492 = local read "out"() -> (w4383:string[])
            n3493 = local read "Total No. of Tests"() -> (w4388:dbl)
            n3494 = Select(t=60.0, s="Run test 3", f=3600.0) -> (s? t:f=w4398:dbl)
            n3495 = Index Array(array=w4444, index #1=1 ("index")) -> (element #1=w4443:string, element #2=w4442:string, element #3=w4441:string, element #4=w4440:string, element #5=w4439:string, element #6=w4438:string)  [unwired: 5 in]
            n3496 = Index Array(array=w4434, index #1=1 ("index")) -> (element #1=w4433:string, element #2=w4432:string, element #3=w4431:string, element #4=w4430:string, element #5=w4429:string, element #6=w4428:string)  [unwired: 5 in]
            n3497 = Index Array(array=w4463, index #1=1 ("index")) -> (element #1=w4462:string, element #2=w4461:string, element #3=w4460:string, element #4=w4459:string, element #5=w4449:string, element #6=w4448:string)  [unwired: 5 in]
            n3498 = Index Array(array=w4383, index #1=1 ("index")) -> (element #1=w4415:string, element #2=w4414:string, element #3=w4413:string, element #4=w4412:string, element #5=w4411:string, element #6=w4410:string)  [unwired: 5 in]
            n3499 = local read "SEN.RUN HRS"() -> (w4386:dbl)
            n3500 = Divide(x=w4390, y=w4398) -> (x/y=w4397:dbl)
            n3501 = Increment(x=w4397) -> (x+1=w4393:dbl)
            n3502 = Number To Decimal String(number=w4393) -> (decimal integer string=→"run hrs":string)  [unwired: 1 in]
            n3503 = Divide(x=w4386, y=3600.0 ("f")) -> (x/y=w4381:dbl)
            n3504 = Round To Nearest(number=w4381) -> (nearest integer value=w4379:dbl)
            n3505 = Number To Decimal String(number=w4379) -> (decimal integer string=w4380:string)  [unwired: 1 in]
            n3506 = Number To Decimal String(number=w4388) -> (decimal integer string=w4389:string)  [unwired: 1 in]
            n3507 = local read "Model No"() -> (w4394:string)
            n3508 = local read "UUID"() -> (w4489:string)
            n3509 = local read "Serial No"() -> (w4493:string)
            n3510 = local read "Secret Key"() -> (w4494:string)
            n3511 = Concatenate Strings("\",\"MachineSerialNumber\":\"" ("string"), w4493) -> (w4497:string)
            n3512 = Concatenate Strings("\",\"ModelNumber\":\"" ("string"), w4394) -> (w4395:string)
            n3513 = Concatenate Strings("\",\"MachineRuntimeHours\":\"" ("string"), w4380) -> (w4498:string)
            n3514 = Concatenate Strings("\",\"MachineRuntimeCycles\":\"", w4389) -> (w4491:string)
            n3515 = Concatenate Strings(w4447, w4443) -> (w4477:string)
            n3516 = Concatenate Strings(w4446, w4433) -> (w4478:string)
            n3517 = Concatenate Strings(w4445, w4415) -> (w4476:string)
            n3518 = Concatenate Strings(w4497, w4395, w4498, w4491) -> (w4500:string)
            n3519 = Concatenate Strings(w4447, w4442) -> (w4474:string)
            n3520 = Concatenate Strings(w4446, w4432) -> (w4473:string)
            n3521 = Concatenate Strings(w4445, w4414) -> (w4475:string)
            n3522 = Concatenate Strings(w4447, w4441) -> (w4469:string)
            n3523 = Concatenate Strings(w4446, w4431) -> (w4470:string)
            n3524 = Concatenate Strings(w4445, w4413) -> (w4468:string)
            n3525 = Concatenate Strings(w4447, w4440) -> (w4466:string)
            n3526 = Concatenate Strings(w4446, w4430) -> (w4465:string)
            n3527 = Concatenate Strings(w4445, w4412) -> (w4467:string)
            n3528 = Concatenate Strings(w4477, w4478, w4476) -> (w4479:string)
            n3529 = Concatenate Strings(w4447, w4439) -> (w4456:string)
            n3530 = Concatenate Strings(w4446, w4429) -> (w4457:string)
            n3531 = Concatenate Strings(w4447, w4438) -> (w4453:string)
            n3532 = Concatenate Strings(w4446, w4428) -> (w4452:string)
            n3533 = Concatenate Strings(w4445, w4411) -> (w4455:string)
            n3534 = Concatenate Strings(w4445, w4410) -> (w4454:string)
            n3535 = Concatenate Strings("{\"SecretKey\":\"", w4494, w4500, "\",\"UUID\" : \"", w4489, "\",\"SensorInformation\":", "[{" ("string")) -> (w4427:string)
            n3536 = Concatenate Strings(w4474, w4473, w4475) -> (w4472:string)
            n3537 = Concatenate Strings(w4469, w4470, w4468) -> (w4471:string)
            n3538 = Concatenate Strings(w4466, w4465, w4467) -> (w4464:string)
            n3539 = Concatenate Strings(w4456, w4457, w4455) -> (w4458:string)
            n3540 = Concatenate Strings(w4453, w4452, w4454) -> (w4451:string)
            n3541 = Concatenate Strings(w4450, w4462, w4479, w4420) -> (w4426:string)
            n3542 = Concatenate Strings(w4450, w4461, w4472, w4420) -> (w4425:string)
            n3543 = Concatenate Strings(w4450, w4460, w4471, w4420) -> (w4424:string)
            n3544 = Concatenate Strings(w4450, w4459, w4464, w4420) -> (w4423:string)
            n3545 = Concatenate Strings(w4450, w4449, w4458, w4420) -> (w4422:string)
            n3546 = Concatenate Strings(w4450, w4448, w4451, "\"}" ("string")) -> (w4421:string)
            n3547 = Concatenate Strings(w4427, w4426, w4425, w4424, w4423, w4422, w4421, "]}" ("string")) -> (w4418:string)
            n3548 = local read "SEN.RUN HRS"() -> (w4385:dbl)
            n3549 = disable-structure shown="Disabled" {
              frame Disabled {
                n3550 = local read "state"() -> (w4504:string[])
                n3551 = Delete From Array(array=w4504, index=0) -> (array with subset deleted=w4502:string[])  [unwired: 1 in, 1 out]
                n3552 = for {
                  N: 6 -> [_]
                  tunnel: w4502 -> [w4515] mode=indexing
                  tunnel: [w4514] -> w4501 mode=indexing
                  n3553 = Equal?(x=w4515, y="Warning") -> (x = y?=w4511:bool)
                  n3554 = Equal?(x=w4515, y="Healthy") -> (x = y?=w4508:bool)
                  n3555 = Select(t="2" ("y"), s=w4511, f="3" ("y")) -> (s? t:f=w4506:string)
                  n3556 = Select(t="1" ("y"), s=w4508, f=w4506) -> (s? t:f=w4514:string)
                }
                "state1" <- w4501
              }
              frame Enabled {
              }
            }
            n3557 = stacked-sequence {
              tunnel: w4418 -> [w4526 _ _]
              tunnel: [_ _ w4542] -> _
              frame #0 {
                (unwired) FALSE ("convert eol (F)")
                w4528 = enum16{"start", "end", "current"}."start" ("pos mode (0:2)")
                n3558 = local read "Path"() -> (w4522:path)
                n3559 = Path To String(path=w4522) -> (string=w4534:string)
                n3560 = Concatenate Strings(w4534, "\\", "Sensor File Name") -> (w4535:string)
                n3561 = local write "standard output 2"(" ") -> ()
                n3562 = String To Path(string=w4535) -> (path=w4525:path)
                n3563 = call <vilib>:"Open_Create_Replace File.vi"("advisory dialog? (display:T)"=FALSE, "function (open:0)"=T25."create or replace", "file path"=w4525) -> ("error out"=w4538:errorcluster, "refnum"=w4537:refnum<file>)  [unwired: 5 in, 2 out]
                n3564 = Set File Position(refnum=w4537, from (0:start)=w4528, error in=w4538) -> (refnum out=w4518:refnum<file>, error out=w4517:errorcluster)  [unwired: 1 in]
                n3565 = Write to Binary File(file (use dialog)=w4518, data=" ", error in=w4517, 5:FALSE ("prepend array or string size? (T)")) -> (refnum out=w4529:refnum<file>, error out=w4530:errorcluster)  [unwired: 2 in, 1 out]
                n3566 = Set File Position(offset (in bytes) (0)=w4528, refnum=w4529, error in=w4530) -> (refnum out=w4521:refnum<file>, error out=w4520:errorcluster)  [unwired: 1 in]
                n3567 = Write to Binary File(file (use dialog)=w4521, data=w4526, error in=w4520, 5:FALSE ("prepend array or string size? (T)")) -> (error out=w4524:errorcluster)  [unwired: 2 in, 2 out]
                n3568 = flat-sequence {
                  tunnel: w4525 -> [w4540]
                  tunnel: w4524 -> [_]
                  frame #0 {
                    n3569 = call <vilib>:"Read Characters From File.vi"("file path (dialog if empty)"=w4540) -> ("character string"=→"Sensor Health JSON string":string)  [unwired: 5 in, 3 out]
                  }
                }
                "SinglePoint  2" <- w4526
              }
              frame #1 {
              }
              frame #2 {
                (unwired) "\"Stored\": true" ("string")
                n3570 = call <vilib>:"System Exec.vi"("run minimized? (F)"=TRUE, "wait until completion? (T)"=TRUE, "working directory"=path "C:/LAB-IQ-NXT", "command line"="C:\\LAB-IQ-NXT\\JPostH.bat") -> ("standard error"=→"Respose From Server 2":string, "standard output"=w4545:string)  [unwired: 4 in, 2 out]
                "standard output 2" <- w4545
                n3571 = Match Pattern(string=w4545, regular expression="JSONH Check String") -> (match substring=w4543:string, offset past match=w4542:i32)  [unwired: 1 in, 2 out]
                n3572 = Equal?(x=w4543, y="JSONH Check String") -> (x = y?=→"Upload \nConfirmed 2":bool)
              }
            }
            n3573 = Divide(x=w4385, y=3600.0 ("f")) -> (x/y=w4378:dbl)
            n3574 = local read "run time"() -> (w4435:string[])
            n3575 = Round To Nearest(number=w4378) -> (nearest integer value=w4377:dbl)
            n3576 = Number To Decimal String(number=w4377) -> (decimal integer string=w4376:string)  [unwired: 1 in]
            n3577 = Index Array(array="Sensor Information", index (col) #1=0 ("disabled index (col)"), index (col) #2=1 ("index (col)"), index (col) #3=2 ("index (col)"), index (col) #4=3 ("index (col)")) -> (element #1=→"Sensor name":string[], element #2=→"model num":string[], element #3=→"run time":string[], element #4=→"state":string[])  [unwired: 4 in]
            n3578 = Insert Into Array(array=w4435, index=1, new element #1=w4376, new element #2=w4376, new element #3=w4376, new element #4=w4376, new element #5=w4376, new element #6=w4376) -> (w4400:string[])
            "run" <- w4400
            n3579 = local read "out"() -> (w4382:string[])
            n3580 = local read "Sensor Information"() -> (w4402:string[][])
            n3581 = Replace Array Subset(array=w4402, new element #1=w4400, index (col) #1=2 ("disabled index (col)"), new element #2=w4382, index (col) #2=3 ("index (col)")) -> (w4401:string[][])  [unwired: 2 in]
            n3582 = local write "Sensor Information"(w4401) -> ()
          }
        }
        n3583 = case shown="True" w4349 {
          frame False {
          }
          frame True {
            n3584 = Equal?(x="FLAG", y=0.0) -> (x = y?=w4366:bool)
            n3585 = case shown="False" w4366 {
              frame False {
                n3586 = Get Date/Time In Seconds() -> (seconds since 1Jan1904=w4372:timestamp)
                n3587 = local read "START 2"() -> (w4370:dbl)
                n3588 = To Double Precision Float(number=w4372) -> (double precision float=w4371:dbl)
                n3589 = Subtract(x=w4371, y=w4370) -> (x-y=→"SENSOR TIME  2":dbl)
              }
              frame True {
                n3590 = Get Date/Time In Seconds() -> (seconds since 1Jan1904=w4374:timestamp)
                n3591 = To Double Precision Float(number=w4374) -> (double precision float=→"START 2":dbl)
                n3592 = local write "FLAG"(100.0 ("FLAG")) -> ()
              }
            }
          }
        }
        n3593 = disable-structure shown="Disabled" {
          disable-tunnel: w4352 -> [w4361 _]
          disable-tunnel: [w4360 _] -> w4351
          frame Disabled {
            n3594 = local read "Json St Flg"() -> (w4359:bool)
            n3595 = case shown="True" w4359 {
              tunnel: w4361 -> [w4362 w4364]
              tunnel: [w4362 w4363] -> w4360
